vi "MGI Defer Panel Updates.vi"(8 "Error In":errorcluster, 10 "Defer Updates?":bool, 11 "VI Reference (Caller)":refnum<vi>) -> (0 "Error Out":errorcluster)   [LabVIEW 2020]
doc: "Defers or Restores Panel Updates for the specified VI.\nThis VI tracks the number of times a defer/restore is made for each VI so that multiple defers must be matched with multiple restores. A Defer or Restore will be attempted even if an error exists on input.\n\nAuthored by Shawn Walpole\nsupport@mooregoodideas.com\nwww.mooregoodideas.com\n\nCopyright (c) 2010, Moore Good Ideas, Inc.\n\nAll rights reserved.\n\nRedistribution and use in source and binary forms, with or without modification, are permitted provided that the following conditions are met:\n\n * Redistributions of source code must retain the above copyright notice, this list of conditions and the following disclaimer.\n * Redistributions in binary form must reproduce the above copyright notice, this list of conditions and the following disclaimer in the documentation and/or other materials provided with the distribution.\n * Neither the name of Moore Good Ideas, Inc. nor the names of its contributors may be used to endorse or promote products derived from this software without specific prior written permission.\n\nTHIS SOFTWARE IS PROVIDED BY THE COPYRIGHT HOLDERS AND CONTRIBUTORS \"AS IS\" AND ANY EXPRESS OR IMPLIED WARRANTIES, INCLUDING, BUT NOT LIMITED TO, THE IMPLIED WARRANTIES OF MERCHANTABILITY AND FITNESS FOR A PARTICULAR PURPOSE ARE DISCLAIMED. IN NO EVENT SHALL THE COPYRIGHT OWNER OR CONTRIBUTORS BE LIABLE FOR ANY DIRECT, INDIRECT, INCIDENTAL, SPECIAL, EXEMPLARY, OR CONSEQUENTIAL DAMAGES (INCLUDING, BUT NOT LIMITED TO, PROCUREMENT OF SUBSTITUTE GOODS OR SERVICES; LOSS OF USE, DATA, OR PROFITS; OR BUSINESS INTERRUPTION) HOWEVER CAUSED AND ON ANY THEORY OF LIABILITY, WHETHER IN CONTRACT, STRICT LIABILITY, OR TORT (INCLUDING NEGLIGENCE OR OTHERWISE) ARISING IN ANY WAY OUT OF THE USE OF THIS SOFTWARE, EVEN IF ADVISED OF THE POSSIBILITY OF SUCH DAMAGE."
uses:
  <userlib>/_MGI/Application Control/MGI VI Reference/MGI Caller's VI Reference.vi
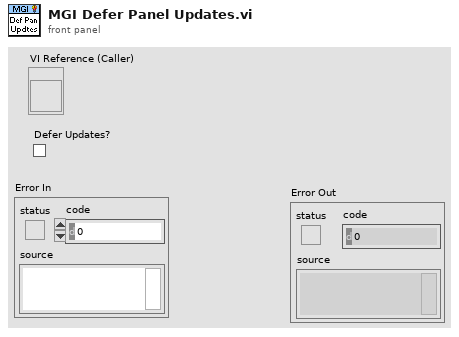
[diagram p1: front panel]
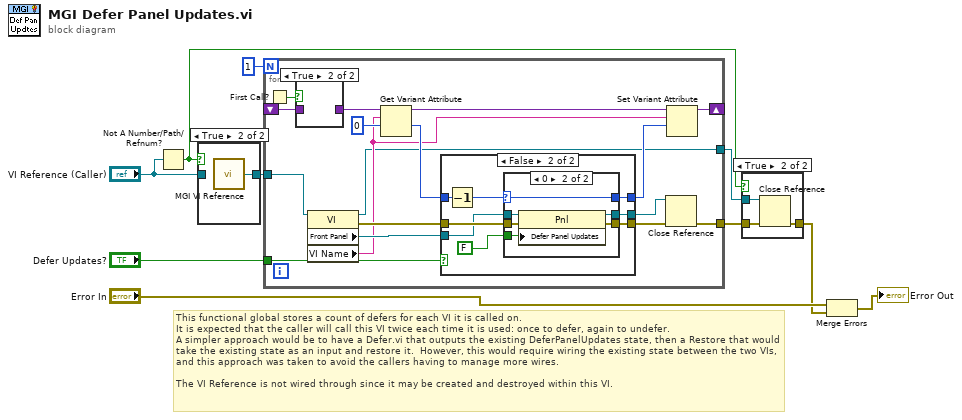
[diagram p0: block diagram]
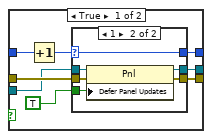
[diagram p3: hidden frame]
diagram:
  # "This functional global stores a count of defers for each VI it is called on.\nIt is expected that the caller will call this VI twice each time it is used: once to defer, again to undefer.\nA simpler approach would be to have a Defer.vi that outputs the existing DeferPanelUpdates state, then a Restore that would take the existing state as an input and restore it.  However, this would require wiring the existing state between the two VIs, and this approach was taken to avoid the callers having to manage more wires.\n\nThe VI Reference is not wired through since it may be created and destroyed within this VI."
  n1 = Not A Number/Path/Refnum?(number/path/refnum="VI Reference (Caller)") -> (NaN/Path/Refnum?=w7:bool)
  n2 = case shown="True" w7 {
    tunnel: "VI Reference (Caller)" -> [w11 _]
    tunnel: [w11 w12] -> w8
    frame False {
    }
    frame True {
      n3 = call-poly <userlib>:"MGI VI Reference.vi"() -> ("Caller's VI Reference"=w12:refnum<vi>)  [unwired: 1 in]
    }
  }
  n4 = for {
    N: 1 -> [_]
    shift-right: [w29] -> _
    shift-left: _ -> [w21]
    tunnel: w8 -> [w14]
    tunnel: "Defer Updates?" -> [w25]
    tunnel: [w13] -> w5
    tunnel: [w15] -> w6
    n5 = First Call?() -> (First Call?: T/F=w22:bool)
    n6 = case shown="True" w22 {
      tunnel: w21 -> [w30 _]
      tunnel: [w30 _] -> w20
      frame False {
      }
      frame True {
      }
    }
    n7 = property class="VI"(reference=w14) -> (reference out=w13:refnum<vi>, error out=w26:errorcluster, "Front Panel"=w23:refnum<vi>, "VI Name"=w18:string)  [unwired: 1 in]
    n8 = Get Variant Attribute(Variant=w20, name=w18, default value (empty Variant)=0) -> (duplicate Variant=w28:variant, value=w24:i32)  [unwired: 1 in, 2 out]
    n9 = case shown="False" w25 {
      tunnel: w26 -> [w38 w55]
      tunnel: w24 -> [w33 w50]
      tunnel: w23 -> [w37 w54]
      tunnel: [w36 w53] -> w17
      tunnel: [w31 w48] -> w19
      tunnel: [w34 w51] -> w16
      frame True {
        n10 = Increment(x=w33) -> (x+1=w32:i32)
        n11 = case shown="1" w32 {
          selector: w32 -> [w39 w42]
          tunnel: w38 -> [w41 w47]
          tunnel: w37 -> [w40 w46]
          tunnel: TRUE -> [_ w45]
          tunnel: [w41 w44] -> w36
          tunnel: [w40 w43] -> w34
          tunnel: [w39 w42] -> w31
          frame Default {
          }
          frame 1 {
            n12 = property class="Pnl"(reference=w46, error in=w47, "Defer Panel Updates"=w45) -> (reference out=w43:refnum<vi>, error out=w44:errorcluster)
          }
        }
      }
      frame False {
        n13 = Decrement(x=w50) -> (x-1=w49:i32)
        n14 = case shown="0" w49 {
          selector: w49 -> [w56 w59]
          tunnel: w55 -> [w58 w64]
          tunnel: w54 -> [w57 w63]
          tunnel: FALSE -> [_ w62]
          tunnel: [w58 w61] -> w53
          tunnel: [w57 w60] -> w51
          tunnel: [w56 w59] -> w48
          frame Default {
          }
          frame 0 {
            n15 = property class="Pnl"(reference=w63, error in=w64, "Defer Panel Updates"=w62) -> (reference out=w60:refnum<vi>, error out=w61:errorcluster)
          }
        }
      }
    }
    n16 = Close Reference(reference=w16, error in (no error)=w17) -> (error out=w15:errorcluster)
    n17 = Set Variant Attribute(Variant=w28, name=w18, value=w19) -> (Variant out=w29:variant)  [unwired: 1 in, 2 out]
  }
  n18 = case shown="True" w7 {
    tunnel: w6 -> [w65 w67]
    tunnel: w5 -> [_ w68]
    tunnel: [w65 w66] -> w2
    frame False {
    }
    frame True {
      n19 = Close Reference(reference=w68, error in (no error)=w67) -> (error out=w66:errorcluster)
    }
  }
  n20 = Merge Errors("Error In", w2) -> (→"Error Out":errorcluster)
